vi "PID 3rd.vi"() -> ()   [LabVIEW 2016]
uses:
  <vilib>/NXT/HiTechnic/HiTechnic Controls/HiTechnic Port.ctl
  <vilib>/NXT/Block Support/NXT_InputPort.ctl
  <vilib>/NXT/Block Support/NXT_OutputPort.ctl
  <vilib>/NXT/Dual Mode Library/Waits/Wait_Num.vi
  <vilib>/NXT/HiTechnic/HiTechnic SubVIs/HiTechnic Angle Sensor Angle.vi
  <vilib>/NXT/Dual Mode Library/prims/inRangeAndCoerce/inRangeAndCoerce_float.vi
  <vilib>/NXT/NXTIO Xnodes/NXTIONodeSubVIs/NXTMoveMotors.vi
  <vilib>/NXT/NXTIO Xnodes/NXTIONodeSubVIs/NXTStopMotors.vi
  <vilib>/NXT/NXTIO Xnodes/AddressXNode/NXTIOAddress.xnode
  <vilib>/NXT/Subs/LVHSConnector.ctl
  <vilib>/NXT/NXTIO Xnodes/NXTIOXNode/NXTIO.xnode
  <vilib>/NXT/LegoClasses/BrickReference/BrickReference.lvclass
panel:
  out "OUTPUT":i32
  out "ERROR 2":i32
  out "Motor Power":dbl
  out "ERROR":dbl
  out "Current Value":dbl
  out "Setpoint":dbl
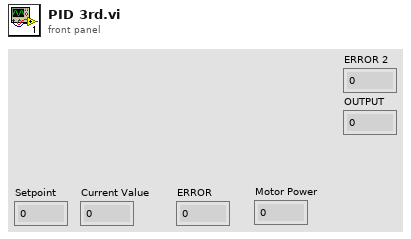
[diagram p1: front panel]
types:
  T1 = typedef "HiTechnic Port.ctl" = cluster{"Port":T2, "MUX Port":u8}
  T2 = typedef "NXT_InputPort.ctl" = u32
  T3 = typedef "LVHSConnector.ctl" = refnum<class "BrickReference.lvclass">
  T4 = typedef "NXT_OutputPort.ctl" = u8
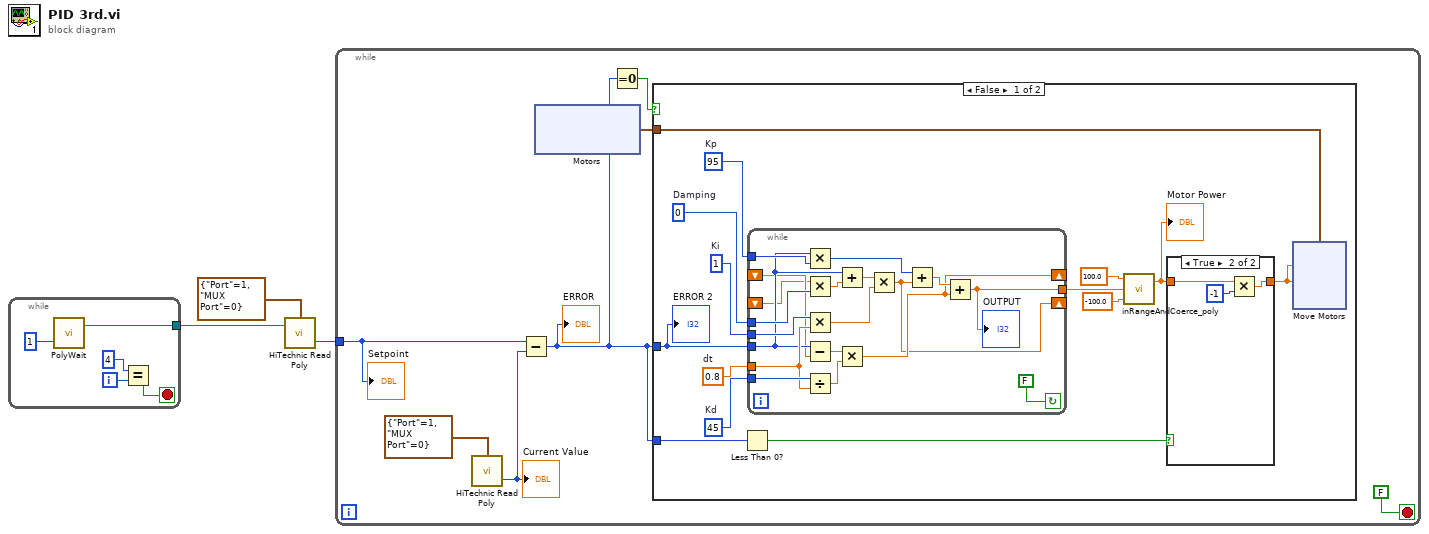
[diagram p0: block diagram]
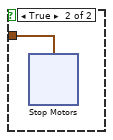
[diagram p3: hidden frame]
diagram:
  n1 = while {
    tunnel: [w5] -> w2
    i -> [w6]
    stop <- w8 stop-if-true
    n2 = call-poly <vilib>:"PolyWait.vi"("Time (1 sec)"=u16 1 ("Duration (500 ms)")) -> ("NXT/EV3"=w5:T3)  [unwired: 3 in]
    n3 = Equal?(x=4, y=w6) -> (x = y?=w8:bool)
  }
  n4 = call-poly <vilib>:"HiTechnic Read Poly.vi"("NXT/EV3"=w2, "Port/MUX"=T1 {"Port"=1, "MUX Port"=0}) -> ("Angle (degrees)"=w1:i32)  [unwired: 1 in, 1 out]
  n5 = while {
    tunnel: w1 -> [w15]
    stop <- FALSE stop-if-true
    n6 = call-poly <vilib>:"HiTechnic Read Poly.vi"("Port/MUX"=T1 {"Port"=1, "MUX Port"=0}) -> ("Angle (degrees)"=w9:i32)  [unwired: 2 in, 1 out]
    "Current Value" <- w9
    n7 = Subtract(x=w15, y=w9) -> (x-y=w13:i32)
    "ERROR" <- w13
    n8 = xnode "Motors"() -> ("Motor"=w12:cluster{"Port":T4, "Port":T4})
    n9 = Equal To 0?(x=w13) -> (x = 0?=w14:bool)
    n10 = case shown="False" w14 {
      tunnel: w13 -> [w30 _]
      tunnel: w13 -> [w29 _]
      tunnel: w12 -> [w19 w62]
      frame False {
        w24 = 0.8  # dt
        w23 = 0  # Damping
        w25 = 45  # Kd
        w26 = 1  # Ki
        w27 = 95  # Kp
        n11 = Less Than 0?(x=w29) -> (x < 0?=w28:bool)
        n12 = while {
          tunnel: w30 -> [w47]
          tunnel: w27 -> [w57]
          tunnel: w26 -> [w55]
          tunnel: w25 -> [w54]
          tunnel: w24 -> [w53]
          tunnel: w23 -> [w56]
          tunnel: [w44] -> w22
          shift-right: [w41] -> _
          shift-left: _ -> [w42]
          shift-right: [w39] -> _
          shift-left: _ -> [w40]
          stop <- FALSE continue-if-true
          n13 = Multiply(x=w47, y=w57) -> (x*y=w52:i32)
          n14 = Multiply(x=w40, y=w56) -> (x*y=w50:dbl)
          n15 = Multiply(x=w55, y=w53) -> (x*y=w51:dbl)
          n16 = Subtract(x=w47, y=w42) -> (x-y=w45:dbl)
          n17 = Divide(x=w54, y=w53) -> (x/y=w46:dbl)
          n18 = Add(x=w47, y=w50) -> (x+y=w49:dbl)
          n19 = Multiply(x=w45, y=w46) -> (x*y=w41:dbl)
          n20 = Multiply(x=w49, y=w51) -> (x*y=w39:dbl)
          n21 = Add(x=w52, y=w39) -> (x+y=w48:dbl)
          n22 = Add(x=w48, y=w41) -> (x+y=w44:dbl)
          "OUTPUT" <- w44
        }
        n23 = call-poly <vilib>:"inRangeAndCoerce_poly.vi"("lower limit"=sgl -100.0, "x"=w22, "upper limit"=sgl 100.0) -> ("coerced(x)"=w17:sgl)  [unwired: 1 out]
        "Motor Power" <- w17
        n24 = case shown="True" w28 {
          tunnel: w17 -> [w58 w60]
          tunnel: [w58 w59] -> w18
          frame False {
          }
          frame True {
            n25 = Multiply(x=w60, y=-1) -> (x*y=w59:sgl)
          }
        }
        n26 = xnode "Move Motors"("Power/Speed 2"=w18, "Power/Speed 1"=w18, "Motors"=w19) -> ()  [unwired: 1 in, 1 out]
        "ERROR 2" <- w30
      }
      frame True {
        n27 = xnode "Stop Motors"("Motors"=w62) -> ()  [unwired: 1 in, 1 out]
      }
    }
    "Setpoint" <- w15
  }
